vi "Main_09b.vi"() -> ()   [LabVIEW 2020]
uses:
  Point.ctl
panel:
  in  "Example 1":string="R 4\nU 4\nL 3\nD 1\nR 4\nD 1\nL 5\nR 2"
  out "Tail Positon count":i32
  in  "Puzzle":string="R 1\nD 1\nL 1\nD 1\nR 2\nL 1\nU 2\nD 1\nU 2\nL 1\nU 1\nL 2\nD 1\nU 2\nL 1\nR 1\nD 1\nL 2\nD 2\nL 2\nR 1\nL 2\nU 2\nR 2\nL 2\nU 2\nL 1\nD 1\nL 2\nU 1\nR 1\nD 2\nL 2\nU 1\nR 1\nD 1\nU 2\nL 1\nD 2\nU 1\nD 1\nR 2\nD 1\nL 2\nD 1\nL 1\nR 1\nD 2\nL 1\nR 2\nD 2\nU 2\nR 2\nD 2\nR 2\nL 2\nD 2\nL 2\nD 1\nU 2\nR 1\nD 2\nL 2\nR 2\nL 1\nD 1\nU 2\nD 1\nR 2\nU 2\nR 2\nD 1\nL 1\nU 2\nD 1\nU 1\nD 2\nU 1\nR 1\nU 2\nD 1\nL 2\nU 1\nL 2\nD 2\nR 1\nU 2\nL 1\nD 2\nR 1\nU 1\nD 1\nL 2\nU 1\nR 1\nD 2\nU 2\nL 1\nU 2\nD 2\nR 1\nU 2\nR 1\nU 2\nR 1\nD 2\nU 1\nD 2\nL 2\nD 2\nL 2\nD 2\nR 1\nU 1\nD 3\nU 1\nR 2\nU 3\nD 1\nU 2\nD 2\nU 2\nD 1\nU 2\nR 2\nL 2\nU 1\nL 3\nD 1\nR 3\nD 3\nR 2\nL 1\nU 3\nD 1\nU 2\nR 2\nD 1\nR 3\nD 2\nR 3\nD 1\nU 3\nL 3\nR 2\nU 3\nL 3\nU 2\nL 3\nD 1\nR 3\nU 3\nR 2\nD 1\nU 3\nR 3\nD 1\nL 2\nD 2\nL 2\nD 3\nR 2\nU 3\nL 3\nD 2\nU 3\nL 2\nU 3\nD 1\nL 1\nD 3\nR 1\nD 3\nU 1\nL 3\nU 1\nD 2\nU 1\nD 1\nU 2\nD 3\nL 1\nU 1\nR 1\nU 3\nD 3\nR 1\nL 2\nR 3\nL 3\nU 1\nD 2\nR 2\nU 2\nD 3\nU 2\nD 3\nL 1\nR 3\nD 3\nR 2\nU 3\nD 3\nL 2\nR 3\nD 3\nR 2\nL 1\nR 3\nD 2\nR 1\nD 3\nL 1\nU 1\nD 2\nR 1\nD 1\nL 1\nR 2\nL 1\nU 1\nL 2\nD 2\nL 2\nD 1\nL 2\nU 3\nD 1\nR 3\nL 2\nR 1\nL 2\nR 3\nU 2\nL 4\nR 3\nL 1\nR 2\nD 2\nL 4\nU 3\nL 1\nD 1\nL 3\nU 2\nL 3\nU 2\nL 1\nR 2\nL 3\nU 1\nD 2\nR 1\nL 4\nR 4\nL 4\nU 2\nD 2\nR 2\nL 2\nU 2\nR 1\nD 3\nL 4\nR 2\nU 1\nL 4\nR 1\nL 1\nD 4\nR 3\nD 1\nR 2\nL 2\nR 3\nL 1\nU 1\nD 3\nU 2\nR 1\nL 1\nD 3\nR 2\nU 2\nR 3\nU 2\nD 1\nR 4\nU 4\nD 3\nU 3\nR 2\nU 1\nL 1\nU 4\nD 1\nR 4\nD 4\nL 3\nU 4\nR 4\nL 1\nR 1\nU 2\nR 4\nD 2\nR 1\nU 2\nL 1\nD 1\nL 3\nR 3\nL 3\nD 3\nL 4\nD 2\nU 2\nD 3\nR 1\nU 1\nD 3\nU 1\nR 3\nD 2\nL 3\nR 2\nD 1\nL 3\nD 3\nU 3\nD 4\nL 2\nU 3\nD 5\nL 2\nD 2\nR 2\nL 3\nD 5\nU 4\nR 1\nD 5\nR 1\nD 1\nL 2\nR 4\nU 2\nD 3\nR 5\nL 2\nR 2\nD 1\nR 2\nU 5\nL 4\nU 5\nD 1\nL 2\nU 2\nR 2\nD 4\nU 3\nL 2\nD 1\nU 4\nL 4\nD 3\nL 3\nD 3\nR 1\nU 1\nR 1\nU 1\nR 2\nD 3\nR 5\nU 1\nD 2\nL 5\nU 5\nL 4\nD 4\nU 4\nL 1\nR 5\nU 2\nL 3\nU 2\nD 3\nL 5\nD 5\nL 2\nU 2\nD 4\nU 3\nD 3\nL 1\nD 2\nR 2\nD 1\nR 4\nL 3\nD 1\nU 4\nL 1\nR 2\nL 4\nD 5\nR 3\nD 1\nL 5\nD 5\nU 3\nR 2\nD 4\nL 2\nR 2\nD 3\nR 3\nU 2\nR 5\nU 4\nR 3\nL 1\nD 2\nU 1\nL 1\nR 2\nU 4\nD 4\nL 1\nR 1\nU 4\nL 3\nU 5\nR 3\nL 4\nD 3\nU 1\nR 4\nU 1\nL 1\nU 3\nR 4\nL 5\nD 1\nU 4\nR 5\nL 1\nR 4\nD 2\nL 6\nD 5\nU 5\nL 5\nR 6\nD 1\nU 2\nR 1\nU 4\nD 6\nL 6\nD 6\nU 6\nD 4\nU 4\nD 1\nU 3\nL 5\nD 6\nR 1\nL 1\nD 2\nL 4\nD 4\nL 4\nR 4\nU 2\nL 3\nD 4\nR 3\nD 4\nU 5\nR 4\nU 1\nR 6\nL 3\nR 2\nU 1\nL 1\nR 2\nD 3\nR 6\nD 6\nU 1\nD 3\nU 4\nD 5\nL 5\nU 3\nD 6\nL 5\nR 5\nU 1\nR 4\nD 2\nL 2\nR 4\nL 5\nR 4\nL 3\nD 5\nR 6\nL 6\nU 1\nR 5\nU 6\nD 2\nR 2\nD 1\nL 6\nU 4\nL 1\nR 5\nL 1\nR 2\nD 1\nL 4\nU 4\nL 1\nR 3\nU 5\nL 2\nD 6\nU 5\nR 6\nD 6\nU 3\nL 3\nU 3\nL 4\nD 5\nU 2\nD 4\nU 5\nR 6\nU 5\nD 2\nU 6\nD 3\nL 3\nD 6\nL 5\nR 2\nD 6\nR 7\nD 3\nL 7\nD 3\nU 2\nR 7\nU 2\nL 6\nR 7\nD 3\nR 7\nU 5\nR 7\nL 5\nR 7\nL 7\nU 4\nD 4\nU 1\nD 3\nU 1\nD 5\nR 3\nU 1\nD 2\nU 1\nL 4\nU 2\nL 6\nD 7\nU 1\nD 4\nU 6\nL 4\nR 4\nD 4\nR 6\nD 7\nR 1\nD 7\nL 4\nR 4\nL 1\nU 1\nR 6\nL 7\nD 7\nL 5\nU 7\nD 3\nL 6\nD 6\nU 4\nR 1\nL 2\nD 4\nR 3\nL 1\nR 7\nD 1\nL 2\nU 1\nD 2\nR 1\nU 3\nD 4\nL 3\nU 6\nL 4\nR 2\nL 1\nU 6\nD 1\nR 5\nU 2\nD 2\nL 7\nU 2\nR 5\nD 2\nR 4\nD 4\nR 3\nL 2\nR 3\nU 7\nL 5\nR 7\nU 2\nL 7\nD 3\nU 6\nD 4\nU 4\nD 6\nU 3\nL 6\nR 4\nD 2\nR 4\nD 2\nR 3\nL 5\nD 1\nU 7\nD 4\nL 4\nU 2\nD 2\nU 7\nL 5\nR 6\nU 8\nL 7\nD 2\nU 1\nR 6\nD 4\nL 4\nR 7\nD 1\nL 6\nD 7\nR 7\nU 3\nL 6\nU 1\nL 8\nD 6\nU 8\nL 7\nU 5\nD 8\nL 2\nD 3\nL 8\nU 1\nD 5\nL 4\nR 6\nD 8\nL 6\nU 5\nR 3\nU 7\nR 6\nU 3\nL 3\nD 4\nR 4\nL 2\nR 6\nD 3\nR 3\nL 8\nU 2\nD 6\nU 3\nD 8\nU 6\nD 4\nU 8\nR 7\nD 2\nU 6\nD 6\nR 1\nU 3\nD 3\nR 1\nU 3\nR 1\nD 7\nL 8\nR 8\nU 7\nR 3\nL 8\nU 2\nL 8\nD 4\nU 4\nR 1\nD 3\nR 4\nU 3\nL 7\nU 2\nR 7\nD 2\nU 4\nD 3\nL 8\nD 5\nL 3\nU 4\nD 6\nL 5\nD 2\nU 1\nR 6\nL 4\nR 6\nU 5\nR 8\nU 8\nD 7\nL 5\nD 2\nL 8\nU 2\nD 1\nR 1\nL 7\nU 4\nR 2\nU 7\nD 6\nR 6\nL 5\nU 8\nD 7\nR 8\nL 8\nD 6\nU 6\nR 1\nD 5\nL 7\nR 8\nL 4\nD 3\nL 2\nU 5\nR 9\nL 8\nD 8\nL 2\nR 4\nL 7\nR 5\nL 1\nR 8\nD 8\nL 4\nU 2\nD 7\nL 7\nD 6\nR 8\nL 3\nD 7\nU 1\nR 6\nD 6\nU 6\nL 9\nD 1\nR 7\nL 5\nR 5\nU 5\nD 4\nL 8\nU 4\nD 8\nR 4\nD 6\nU 3\nD 7\nL 5\nD 6\nR 9\nU 4\nR 6\nL 3\nU 4\nD 9\nL 7\nR 5\nD 9\nL 6\nU 7\nL 7\nR 4\nD 5\nR 7\nL 5\nR 3\nU 8\nL 6\nU 5\nL 9\nR 8\nU 4\nD 2\nL 4\nD 7\nR 7\nD 4\nL 4\nU 2\nL 3\nR 1\nD 3\nU 6\nR 1\nU 8\nR 2\nL 4\nD 3\nL 5\nU 4\nR 7\nL 2\nR 7\nL 9\nD 9\nU 5\nL 4\nU 1\nD 1\nU 6\nD 1\nL 6\nD 7\nU 5\nD 9\nR 9\nD 5\nU 9\nL 3\nR 5\nD 10\nR 1\nU 7\nD 6\nL 3\nU 5\nR 1\nD 5\nR 8\nU 3\nL 1\nD 2\nR 1\nL 6\nR 8\nD 9\nU 9\nD 4\nR 1\nU 8\nL 5\nU 4\nD 7\nL 1\nR 4\nL 6\nD 4\nR 5\nD 1\nR 10\nD 5\nR 7\nU 6\nR 5\nU 2\nL 8\nR 1\nU 3\nL 5\nU 4\nL 3\nD 3\nU 6\nD 10\nL 3\nD 7\nL 5\nD 4\nU 6\nR 9\nU 5\nD 5\nR 2\nL 7\nU 8\nD 5\nR 9\nL 6\nR 8\nU 9\nL 4\nR 10\nD 10\nL 9\nR 8\nL 4\nR 5\nL 9\nD 1\nL 3\nR 9\nU 2\nL 5\nR 2\nU 1\nR 4\nD 10\nU 3\nD 8\nL 9\nD 8\nL 5\nD 4\nU 2\nL 8\nR 5\nU 4\nD 1\nL 4\nU 7\nD 9\nR 3\nD 7\nR 9\nL 6\nR 6\nU 8\nL 10\nU 5\nD 4\nR 5\nL 6\nD 7\nL 10\nR 1\nL 9\nU 6\nD 9\nR 7\nL 7\nD 6\nU 6\nR 1\nD 7\nL 1\nR 9\nD 9\nR 3\nL 5\nD 4\nR 3\nL 5\nD 11\nU 1\nR 6\nD 8\nR 4\nD 3\nR 9\nU 3\nD 8\nU 7\nR 2\nU 10\nR 4\nL 4\nD 10\nR 8\nU 11\nR 7\nD 7\nR 9\nD 11\nU 6\nR 7\nD 10\nL 4\nD 5\nL 7\nD 3\nL 4\nD 4\nU 4\nR 3\nL 9\nD 4\nL 8\nU 5\nR 7\nL 2\nD 4\nR 11\nU 10\nD 3\nR 8\nD 3\nR 10\nL 8\nU 6\nR 4\nD 10\nR 7\nD 3\nR 2\nU 1\nD 5\nL 8\nU 2\nR 1\nU 8\nR 11\nL 3\nU 10\nL 5\nD 3\nL 6\nU 10\nL 11\nD 4\nL 5\nD 1\nL 4\nD 1\nL 3\nR 7\nU 7\nR 4\nL 1\nU 10\nD 11\nL 1\nR 1\nU 9\nD 6\nL 9\nD 1\nL 4\nD 11\nL 5\nU 2\nL 5\nD 8\nU 10\nD 5\nU 10\nL 8\nR 11\nD 10\nU 11\nR 4\nU 6\nD 11\nR 1\nL 4\nU 12\nL 8\nU 12\nD 4\nL 7\nU 7\nL 8\nD 3\nU 1\nL 12\nD 5\nU 3\nD 6\nR 7\nU 1\nD 12\nR 6\nU 3\nD 3\nR 12\nU 5\nR 3\nU 8\nL 6\nR 6\nU 3\nL 4\nD 8\nL 5\nD 12\nU 1\nL 9\nR 4\nL 1\nD 6\nU 9\nL 5\nR 3\nL 9\nD 8\nR 6\nD 3\nU 6\nL 1\nD 7\nU 5\nD 1\nL 11\nR 7\nD 11\nL 3\nU 6\nR 9\nD 12\nR 11\nL 5\nR 8\nL 2\nU 10\nR 6\nU 10\nL 9\nU 1\nL 1\nR 8\nL 7\nR 3\nU 4\nL 3\nR 8\nL 9\nR 11\nL 9\nD 11\nU 1\nL 12\nR 6\nL 3\nR 3\nD 12\nU 9\nL 9\nD 8\nR 4\nL 7\nR 1\nU 2\nR 4\nU 4\nR 11\nU 7\nD 11\nU 3\nD 6\nU 7\nL 2\nD 4\nU 9\nR 3\nL 8\nR 9\nL 4\nR 5\nL 7\nD 3\nR 8\nL 6\nU 10\nR 3\nL 6\nD 8\nU 3\nD 9\nL 1\nU 13\nR 12\nL 13\nR 2\nU 8\nR 1\nD 11\nR 5\nL 4\nU 5\nL 3\nD 13\nU 2\nD 1\nU 2\nL 9\nD 3\nR 6\nU 13\nL 3\nU 5\nR 2\nD 2\nL 5\nU 4\nR 6\nD 1\nU 9\nL 7\nR 11\nU 10\nD 12\nR 10\nU 7\nR 5\nL 2\nR 13\nL 13\nD 3\nR 7\nU 1\nL 1\nD 2\nL 9\nU 12\nD 7\nU 13\nL 12\nU 13\nD 7\nU 7\nD 8\nL 2\nU 6\nD 2\nU 6\nL 8\nU 4\nD 11\nU 11\nL 11\nR 10\nL 10\nR 6\nD 13\nU 2\nL 7\nU 8\nD 1\nR 6\nL 7\nR 9\nL 8\nR 9\nL 6\nR 7\nD 12\nR 11\nL 8\nR 1\nD 5\nR 5\nL 10\nU 6\nL 8\nD 9\nL 5\nU 4\nD 12\nU 8\nL 13\nU 6\nD 10\nR 5\nL 13\nD 7\nL 13\nR 5\nL 10\nD 13\nL 9\nR 3\nD 8\nU 9\nD 10\nU 10\nD 7\nL 5\nR 5\nD 9\nL 7\nR 10\nD 13\nR 1\nU 2\nR 6\nU 14\nR 10\nD 6\nU 13\nD 14\nU 5\nD 1\nU 8\nR 4\nU 9\nR 13\nL 4\nD 2\nR 8\nU 2\nD 12\nU 3\nR 6\nU 6\nD 11\nR 7\nL 12\nR 9\nU 7\nD 1\nR 14\nL 11\nU 4\nD 13\nU 5\nL 7\nR 14\nL 1\nU 6\nD 3\nL 1\nU 13\nD 8\nU 14\nD 5\nU 14\nL 1\nR 1\nD 5\nU 7\nL 8\nR 6\nU 1\nD 2\nR 14\nU 13\nL 10\nU 8\nD 13\nU 6\nR 2\nD 4\nR 6\nU 7\nD 10\nL 6\nU 5\nL 3\nD 9\nU 13\nD 8\nU 3\nR 3\nL 12\nD 5\nR 8\nU 7\nR 11\nU 6\nD 7\nR 13\nU 1\nD 9\nU 10\nD 3\nL 5\nR 12\nL 4\nD 13\nR 7\nD 12\nR 11\nD 9\nR 5\nU 13\nR 3\nD 4\nU 10\nR 3\nU 6\nL 4\nR 1\nU 4\nL 9\nD 11\nU 5\nD 3\nU 13\nD 1\nL 1\nD 13\nL 2\nR 9\nL 4\nR 2\nU 9\nD 9\nU 12\nL 14\nR 2\nL 9\nR 5\nU 2\nD 3\nR 13\nU 5\nD 1\nU 15\nR 6\nD 14\nR 8\nL 9\nD 14\nL 6\nR 8\nU 14\nR 11\nL 3\nD 15\nU 5\nR 1\nL 7\nR 12\nD 1\nR 4\nD 13\nU 9\nD 2\nL 3\nU 10\nR 10\nD 2\nR 6\nU 13\nD 7\nR 5\nU 5\nL 12\nU 6\nR 1\nL 7\nU 9\nD 15\nL 8\nU 9\nL 5\nR 3\nL 9\nU 6\nL 11\nD 8\nL 11\nD 13\nU 3\nR 6\nD 2\nL 10\nR 15\nU 2\nD 8\nR 6\nD 6\nL 8\nD 7\nU 2\nD 14\nU 4\nR 6\nD 15\nL 12\nR 4\nD 3\nU 7\nD 10\nL 8\nU 7\nR 10\nU 11\nD 2\nR 10\nD 10\nU 13\nR 8\nL 2\nU 12\nR 9\nU 12\nR 5\nU 10\nL 6\nR 3\nD 10\nL 10\nU 6\nL 4\nR 3\nD 9\nR 15\nD 14\nL 11\nR 5\nU 2\nR 14\nL 15\nR 3\nD 3\nL 4\nU 10\nD 14\nL 9\nD 5\nL 16\nU 12\nL 4\nD 15\nL 10\nR 14\nD 4\nR 12\nL 7\nU 5\nR 3\nL 6\nU 16\nL 5\nU 8\nD 8\nL 6\nD 3\nU 14\nR 1\nL 13\nU 4\nD 11\nR 5\nL 11\nD 7\nR 1\nL 14\nU 10\nL 5\nD 15\nU 14\nL 4\nD 7\nU 3\nR 1\nU 2\nR 3\nD 16\nU 7\nR 7\nD 13\nR 7\nD 5\nU 7\nR 16\nU 4\nL 3\nR 9\nU 1\nD 2\nR 5\nD 3\nU 8\nR 5\nL 13\nU 13\nL 2\nR 9\nL 14\nD 10\nR 1\nU 1\nR 14\nU 14\nR 2\nL 1\nR 12\nL 1\nD 6\nR 2\nD 7\nR 11\nL 5\nD 8\nR 15\nD 12\nR 12\nL 8\nD 10\nR 2\nD 12\nU 15\nL 9\nD 4\nU 3\nL 8\nD 3\nU 9\nD 16\nL 2\nU 14\nR 15\nD 14\nU 12\nD 6\nU 14\nR 11\nD 12\nR 2\nU 13\nL 2\nR 1\nD 6\nU 13\nD 15\nU 1\nR 14\nL 16\nD 8\nR 13\nL 14\nR 3\nD 8\nL 6\nR 16\nD 6\nL 13\nR 2\nL 11\nD 2\nU 1\nR 15\nL 9\nU 1\nR 12\nL 9\nD 7\nL 8\nU 2\nL 14\nR 7\nU 8\nD 15\nR 8\nD 13\nL 15\nR 11\nD 17\nU 2\nR 14\nL 9\nU 11\nD 6\nU 4\nD 8\nU 16\nD 5\nL 3\nD 11\nL 7\nU 11\nL 4\nD 5\nL 5\nD 2\nU 8\nR 17\nD 17\nU 12\nR 4\nL 13\nR 15\nL 10\nU 2\nL 10\nR 6\nD 1\nU 6\nL 3\nD 8\nR 4\nD 1\nL 4\nD 13\nR 1\nU 3\nL 1\nU 9\nD 13\nU 2\nD 13\nR 6\nD 8\nR 6\nD 13\nR 4\nD 10\nL 10\nU 8\nD 1\nR 6\nU 14\nR 3\nL 10\nU 15\nL 11\nU 13\nL 4\nU 5\nL 16\nR 16\nU 11\nR 14\nD 7\nU 5\nR 9\nL 5\nU 12\nR 16\nU 10\nD 5\nR 17\nL 3\nD 5\nU 13\nR 3\nU 3\nL 14\nU 1\nL 8\nR 2\nD 3\nU 9\nD 7\nL 1\nD 5\nR 16\nD 12\nR 1\nU 2\nL 16\nU 3\nR 18\nD 11\nR 3\nL 17\nR 7\nL 6\nD 13\nL 5\nR 12\nD 3\nU 1\nL 1\nU 5\nL 8\nR 11\nL 13\nD 14\nR 17\nD 17\nL 2\nU 7\nD 18\nR 3\nD 2\nU 6\nD 9\nR 3\nU 3\nR 5\nD 16\nR 9\nD 13\nU 8\nD 17\nR 4\nL 6\nR 7\nD 2\nR 15\nU 10\nR 15\nD 6\nL 8\nR 17\nD 5\nL 9\nU 18\nD 10\nU 3\nL 6\nU 10\nD 10\nU 16\nR 6\nD 18\nU 10\nD 8\nU 14\nR 3\nU 14\nL 16\nR 3\nD 5\nL 2\nR 4\nD 9\nL 13\nR 17\nL 8\nD 2\nR 16\nD 18\nL 11\nD 15\nU 5\nD 7\nU 14\nD 13\nU 7\nL 13\nD 13\nR 1\nD 15\nR 11\nL 1\nU 6\nD 14\nL 6\nU 8\nD 15\nR 8\nL 12\nD 17\nR 8\nL 17\nD 16\nR 9\nD 19\nU 4\nR 9\nU 10\nL 3\nU 3\nD 5\nR 2\nU 6\nL 16\nD 8\nR 4\nL 16\nR 15\nU 6\nL 8\nD 6\nL 6\nR 1\nL 8\nD 13\nL 1\nU 7\nR 16\nL 16\nU 1\nL 18\nD 16\nL 8\nU 2\nD 1\nR 2\nD 10\nU 8\nD 2\nR 18\nU 14\nD 15\nR 15\nU 3\nD 1\nU 17\nL 17\nD 15\nL 14\nR 6\nL 18\nU 19\nL 6\nU 17\nL 1\nD 2\nU 17\nR 11\nL 3\nR 3\nL 12\nU 1\nL 9\nU 13\nD 15\nU 12\nR 1\nL 5\nD 17\nL 14\nD 13\nL 2\nD 10\nU 5\nR 13\nL 19\nD 1\nR 12\nU 17\nR 15\nD 19\nU 12\nD 16\nR 2\nU 3\nR 15\nL 13\nU 11\nD 19\nR 10\nD 19\nL 2\nU 12\nR 5\nL 13\nU 13\nR 1\nD 11\nR 17\nD 7\nU 4\nD 14\nL 13\nR 8\nL 8\nD 8"
  in  "Example 2":string="R 5\nU 8\nL 8\nD 3\nR 17\nD 10\nL 25\nU 20"
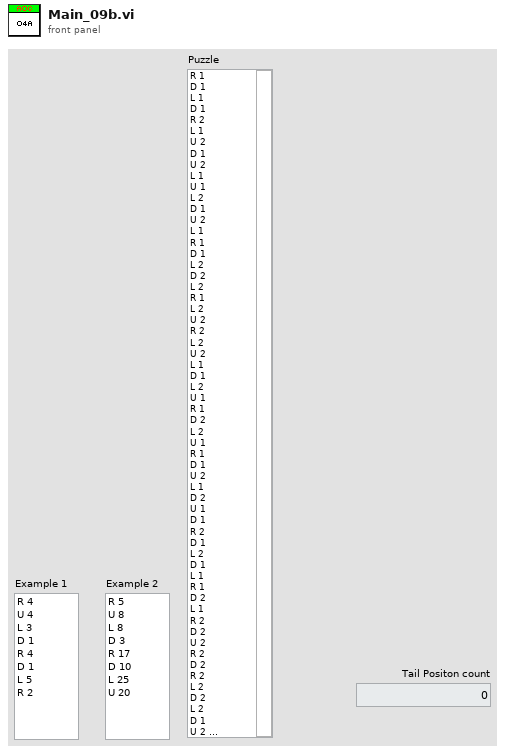
[diagram p1: front panel]
types:
  T1 = typedef "Point.ctl" = cluster{"X":i32, "Y":i32}
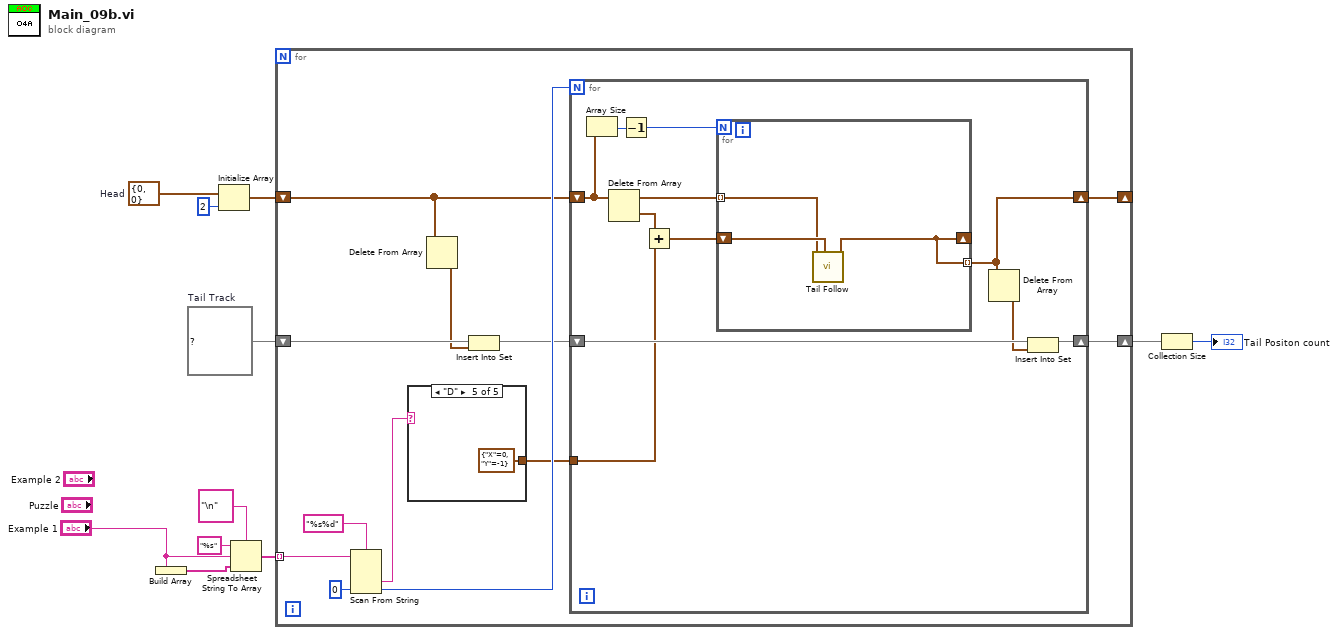
[diagram p0: block diagram]
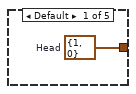
[diagram p2: hidden frame]
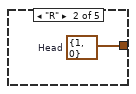
[diagram p3: hidden frame]
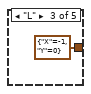
[diagram p4: hidden frame]
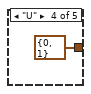
[diagram p5: hidden frame]
diagram:
  w3 = T1 {"X"=0, "Y"=0}  # Head
  w7 = set{T1} {}  # Tail Track
  n1 = Build Array("Example 1") -> (w11:string[])
  n2 = Initialize Array(w3, 2 ("dimension size")) -> (w2:T1[])
  n3 = Spreadsheet String To Array(delimiter (Tab)="\n", format string="%s", spreadsheet string="Example 1", array type (2D Dbl)=w11) -> (array=w8:string[])
  n4 = for {
    tunnel: w8 -> [w22] mode=indexing
    shift-right: [w18] -> w6
    shift-left: w7 -> [w16]
    shift-right: [w12] -> _
    shift-left: w2 -> [w14]
    n5 = Scan From String(format string="%s%d", input string=w22, default 2=0 ("default value 2")) -> (output 1=w21:string, output 2=w19:i32)  [unwired: 3 in, 3 out]
    n6 = case shown="\"D\"" w21 {
      tunnel: [w38 w39 T1 {"X"=-1, "Y"=0} ("Head") T1 {"X"=0, "Y"=1} ("Head") T1 {"X"=0, "Y"=-1} ("Head")] -> w17
      frame Default {
        w38 = T1 {"X"=1, "Y"=0}  # Head
      }
      frame "R" {
        w39 = T1 {"X"=1, "Y"=0}  # Head
      }
      frame "L" {
      }
      frame "U" {
      }
      frame "D" {
      }
    }
    n7 = Delete From Array(array=w14) -> (deleted portion=w13:T1)  [unwired: 2 in, 1 out]
    n8 = Insert Into Set(10:w13, 11:w16) -> (3:w15:set{T1})  [unwired: 1 out]
    n9 = for {
      N: w19 -> [_]
      shift-right: [w33] -> w18
      shift-left: w15 -> [w34]
      tunnel: w17 -> [w28]
      shift-right: [w25] -> w12
      shift-left: w14 -> [w30]
      n10 = Array Size(array=w30) -> (size(s)=w32:i32)
      n11 = Delete From Array(array=w30) -> (deleted portion=w27:T1, array with subset deleted=w29:T1[])  [unwired: 2 in]
      n12 = Decrement(x=w32) -> (x-1=w31:i32)
      n13 = Add(x=w27, y=w28) -> (x+y=w26:T1)
      n14 = for {
        N: w31 -> [_]
        shift-right: [w35] -> _
        shift-left: w26 -> [w37]
        tunnel: w29 -> [w36] mode=indexing
        tunnel: [w35] -> w25 mode=indexing
        n15 = call "Tail Follow.vi"("Head"=w37, "Tail"=w36) -> ("Tail Out"=w35:T1)  [unwired: 9 in]
      }
      n16 = Delete From Array(array=w25) -> (deleted portion=w24:T1)  [unwired: 2 in, 1 out]
      n17 = Insert Into Set(10:w24, 11:w34) -> (3:w33:set{T1})  [unwired: 1 out]
    }
  }
  n18 = Collection Size(1:w6) -> (0:→"Tail Positon count":i32)
